vi "Initialize Hardware.vi"(8 "error in (no error)":errorcluster, 9 "DAQ Type":enum16{"Hardware", "Simulation"}(ring), 10 "Instrument Setting":T1={"Connection"={"Ref"=variant(u32 9600), "Serial"={"Baud Rate"=4, "Parity"=0, "Data Bits"=8, "Flow Control"=4}}, "Ouput Imp"={"User-Defined Impedance (50 Ohms)"=0.0, "Impedance (0: 50 Ohms)"=8}} {"Ouput Imp"."Impedance (0: 50 Ohms)" items=["None", "Odd", "Even", "Mark", "Space"]; "Ouput Imp"."User-Defined Impedance (50 Ohms)" format="%.2f"; "Connection"."Serial"."Flow Control" items=["None", "XON/XOFF", "RTS/CTS", "XON/XOFF & RTS/CTS", "DTR/DSR", "XON/XOFF & DTR/DSR"]; "Connection"."Serial"."Data Bits" items=["7"=7, "8"=8]; "Connection"."Serial"."Parity" items=["None", "Odd", "Even", "Mark", "Space"]; "Connection"."Serial"."Baud Rate" items=["300"=300, "600"=600, "1200"=1200, "2400"=2400, "4800"=4800, "9600"=9600, "19200"=19200]}, 11 "Agilent 33210A in":refnum<class "Agilent 33210A.lvclass">) -> (0 "error out":errorcluster, 3 "Agilent 33210A out":refnum<class "Agilent 33210A.lvclass">)   [LabVIEW 2016, in "Func Generator.lvlib" / "Agilent 33210A.lvclass"]
uses:
  Agilent 33210A.lvclass
  Instrument Setting.ctl
  Agilent 33210A.lvclass/Agilent 33210A.ctl
  <instrlib>/Agilent 33XXX Series/Agilent 33XXX Series.lvlib
  Func Generator.lvlib
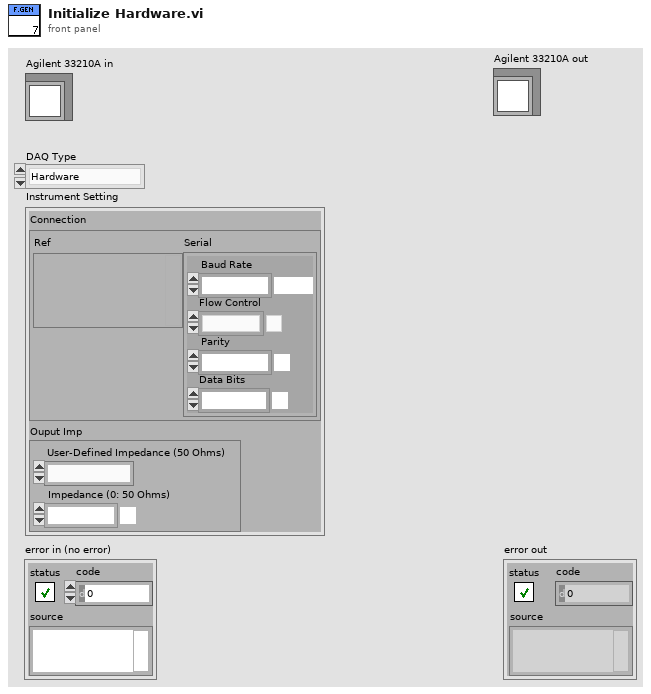
[diagram p1: front panel]
types:
  T1 = typedef "Func Generator.lvlib/Instrument Setting.ctl" = cluster{"Connection":cluster{"Ref":variant, "Serial":cluster{"Baud Rate":u32, "Parity":u16, "Data Bits":u16, "Flow Control":u16}}, "Ouput Imp":cluster{"User-Defined Impedance (50 Ohms)":dbl, "Impedance (0: 50 Ohms)":u16}}
  T2 = cluster{"Baud Rate":u32, "Parity":u16, "Data Bits":u16, "Flow Control":u16}
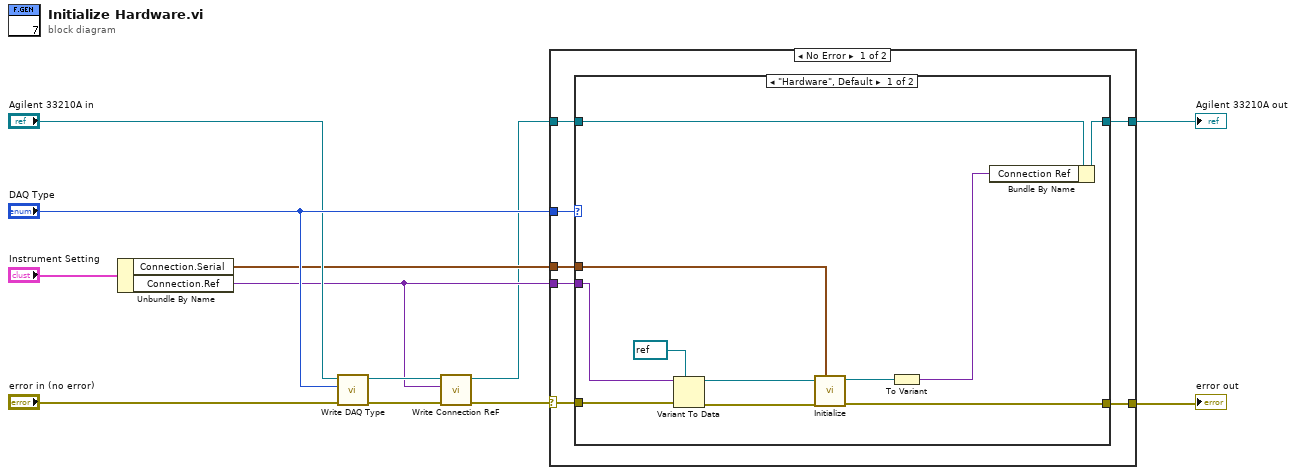
[diagram p0: block diagram]
diagram:
  n1 = Unbundle By Name("Instrument Setting") -> ("Connection.Serial"=w2:T2, "Connection.Ref"=w3:variant)
  n2 = call-dynamic "Write DAQ Type.vi"("error in (no error)"="error in (no error)", "DAQ Type"="DAQ Type", "Agilent 33210A in"="Agilent 33210A in") -> ("error out"=w11:errorcluster, "Agilent 33210A out"=w8:refnum<class "Agilent 33210A.lvclass">)  [unwired: 7 in]
  n3 = call-dynamic "Write Connection ReF.vi"("error in (no error)"=w11, "Connection Ref"=w3, "Agilent 33210A in"=w8) -> ("error out"=w9:errorcluster, "Agilent 33210A out"=w1:refnum<class "Agilent 33210A.lvclass">)  [unwired: 7 in]
  n4 = case shown="No Error" w9 {
    selector: w9 -> [w18 w33]
    tunnel: w3 -> [w17 _]
    tunnel: w1 -> [w16 w34]
    tunnel: "DAQ Type" -> [w19 _]
    tunnel: [w15 w34] -> w6
    tunnel: [w14 w33] -> w5
    tunnel: w2 -> [w13 _]
    frame No Error {
      n5 = case shown="\"Hardware\", Default" w19 {
        tunnel: w18 -> [w29 w31]
        tunnel: w17 -> [w28 _]
        tunnel: w16 -> [w25 w32]
        tunnel: [w23 w32] -> w15
        tunnel: [w24 w31] -> w14
        tunnel: w13 -> [w21 _]
        frame "Hardware", Default {
          n6 = Variant To Data(error in=w29, type=refnum<visa-resource-name> refnum ("VISA resource name"), Variant=w28) -> (data=w26:refnum<visa-resource-name>, error out=w27:errorcluster)
          n7 = call <instrlib>:"Initialize.vi"("Serial Configuration"=w21, "error in (no error)"=w27, "VISA resource name"=w26) -> ("error out"=w24:errorcluster, "VISA resource name out"=w22:refnum<visa-resource-name>)  [unwired: 7 in]
          n8 = To Variant(anything=w22) -> (Variant=w20:variant)
          n9 = Bundle By Name(cluster=w25, "Connection Ref"=w20) -> (w23:refnum<class "Agilent 33210A.lvclass">)
        }
        frame "Simulation" {
        }
      }
    }
    frame Error {
    }
  }
  "error out" <- w5
  "Agilent 33210A out" <- w6
